vi "Assignment1_1.vi"() -> ()   [LabVIEW 2025]
panel:
  out "Digital_Code":ext
  in  "Resolution(bits)":i32
  in  "Voltage_Range(V)":dbl
  in  "Analog_Data(V)":dbl
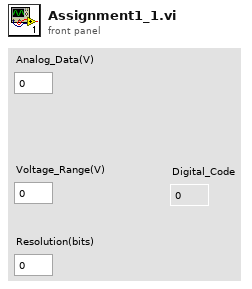
[diagram p1: front panel]
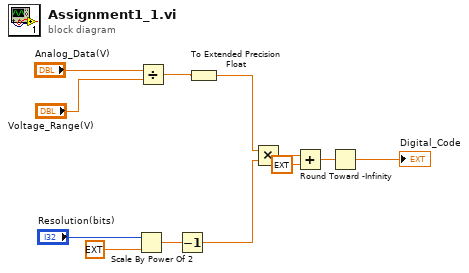
[diagram p0: block diagram]
diagram:
  n1 = Scale By Power Of 2(n="Resolution(bits)", x=ext 1.0) -> (x*2^n=w11:ext)
  n2 = Divide(x="Analog_Data(V)", y="Voltage_Range(V)") -> (x/y=w9:dbl)
  n3 = Decrement(x=w11) -> (x-1=w10:ext)
  n4 = To Extended Precision Float(1:w9) -> (0:w8:ext)
  n5 = Multiply(x=w8, y=w10) -> (x*y=w4:ext)
  n6 = Add(x=w4, y=ext 0.5) -> (x+y=w2:ext)
  n7 = Round Toward -Infinity(1:w2) -> (0:→"Digital_Code":ext)
